vi "enable_channel_ASIC_mezzanine_NEW.vi"(4 "Clip_sel_b":u32, 5 "maj/sum":bool, 6 "Ib_clipVb":u32, 7 "Att gain":u32=4095, 8 "error in":errorcluster, 9 "Channel":u32, 10 "id_in":i32, 11 "connection ID":refnum<k5>) -> (0 "error out":errorcluster, 1 "id_out":i32, 3 "connection ID out":refnum<k5>)   [LabVIEW 2012]
doc: "This VI sends a command to the Integration Board and provides the received data when necessary."
panel:
  out "written data":u32=72
  out "data out serial":string
  out "data read value":u32=72
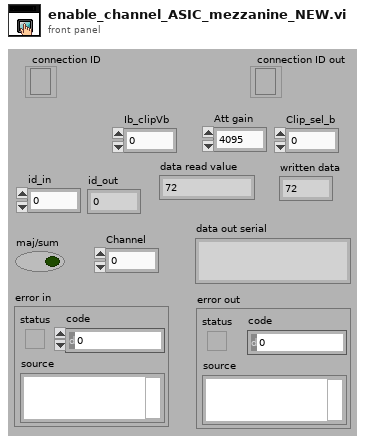
[diagram p1: front panel]
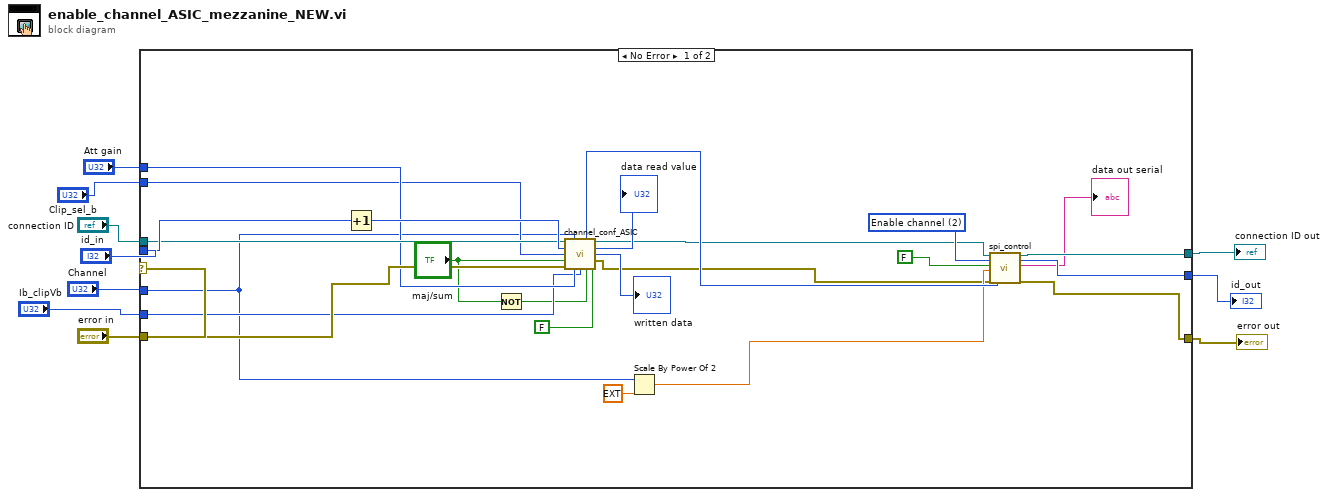
[diagram p0: block diagram]
diagram:
  n1 = case shown="No Error" "error in" {
    tunnel: "id_in" -> [w29 w35]
    tunnel: "error in" -> [w27 w36]
    tunnel: "connection ID" -> [w28 w37]
    tunnel: [w25 w36] -> w8
    tunnel: [w26 w37] -> w7
    tunnel: "Channel" -> [w19 _]
    tunnel: [w24 w35] -> w5
    tunnel: "Att gain" -> [w22 _]
    tunnel: "Ib_clipVb" -> [w21 _]
    tunnel: "Clip_sel_b" -> [w20 _]
    frame No Error {
      w32 = u16 2 items=["Attenuation", "Clipping", "Enable channel", "Delay line", "ASIC"] ("Device")
      n2 = Increment(x=w29) -> (x+1=w34:i32)
      n3 = Not(x="maj/sum") -> (.not. x?=w15:bool)
      n4 = call "channel_conf_ASIC.vi"("connection ID"=w28, "Ring"=w19, "Id in"=w34, "Clip_sel_b"=w20, "CompBuf_en_b"="maj/sum", "error out"=w27, "Att gain"=w22, "Ib_ClipVb"=w21, "Clip_en_b"=w15, "Att_en_b"=FALSE) -> ("Id out"=w33:i32, "connection ID out"=w11:refnum<k5>, "data read value"=→"data read value":u32, "written data"=→"written data":u32, "error out 2"=w12:errorcluster)  [unwired: 1 in]
      n5 = Scale By Power Of 2(n=w19, x=ext 1.0) -> (x*2^n=w13:ext)
      n6 = call "spi_control.vi"("connection ID"=w11, "Device"=w32, "Read/#write"=FALSE, "Data"=w13, "error in"=w12, "Id in"=w33) -> ("connection ID out"=w26:refnum<k5>, "Id out"=w24:i32, "data out serial"=→"data out serial":string, "error out 2"=w25:errorcluster)  [unwired: 6 in, 4 out]
    }
    frame Error {
    }
  }
  "error out" <- w8
  "connection ID out" <- w7
  "id_out" <- w5
